vi "Sequencer.vi"() -> ()   [LabVIEW 2014]
uses:
  <vilib>/gmath/statdist.llb/Poisson Random.vi
  <vilib>/Analysis/NI_AALPro.lvlib
  <vilib>/gmath/NI_Gmath.lvlib
panel:
  in  "Ion":bool
  in  "Protect":bool
  out "PMT":dbl=70.0 format="%.1f"
  in  "Experiment":bool
  in  "Pumping":bool
  in  "Detection":bool
  in  "Cooling":bool
  out "History":variant
  in  "Count or State":i16(ring) items=["Count", "State"]
  in  "Channel":string(combo)="c1+c2+c3+c4"
  in  "Device":string(combo)="PMT"
  in  ">":dbl=1.0
  in  "Fit":bool
  out "Peak":u32
  out "Histogram":cluster{"Axis":dbl[], "Histogram":i32[]}(graph)
  in  "Data Chapter":i16(ring) items=["All", "Ion[2]"]
  out "Average Plot":cluster{dbl, dbl}(graph)
  in  "Clear":bool
  in  "Sweep":bool
  in  "Data":bool
  out "data file":string
  in  "Sequence":string
  in  "Chapter (us)":string
  in  "Sequence File":path=path "E:/Data/Sequence/Cooling.seq"
  in  "Repeats":u32=100
  in  "Compile":bool
  in  "Send":bool
  in  "Port":refnum<visa-resource-name>="COM5"
  in  "Trigger":bool
  in  "Save":bool
  out "Item Function":refnum<vi>
  in  "Set":bool
  in  "Item":string(combo)="Time"
  out "SequenceNames":string[](array[string])
  in  "Parameter":u16(ring) items=["Segment", "Frequency", "Duration", "Amplitude", "Phase", "Gap"]
  in  "Scan":bool
  out "Value":dbl=1.0 format="%.4f"
  in  "Step":dbl=1.0 format="%.4f"
  in  "End":dbl=1.0 format="%.3f"
  in  "Start":dbl=1.0 format="%.3f"
  out "Counts":u32[](array[numeric])
  out "CompiledSequence":string="#DopplerCooling\r\n0.9 10100000 00000000 00000000\r\n\r\n#Pump\r\n0.3 01000000 00000000 00000000\r\n\r\n#Pulsed\r\n0.2 00100000 00000000 00000000\r\n0.4 00000100 00000000 00000000\r\n0.2 00000000 10000000 00000000\r\n0.2 01000000 00000000 01000000\n"
  out "ChapterNames":string[](array[string])
  out "ChapterPositions":u32[](array[numeric])
  out "Durations Backup":dbl[](array[numeric])
  out "Durations":dbl[](array[numeric])
  in  "Period (ns)":dbl=5.0
  out "States":string[](array[string])
  in  "Sequencer":bool
  out "Clock":string
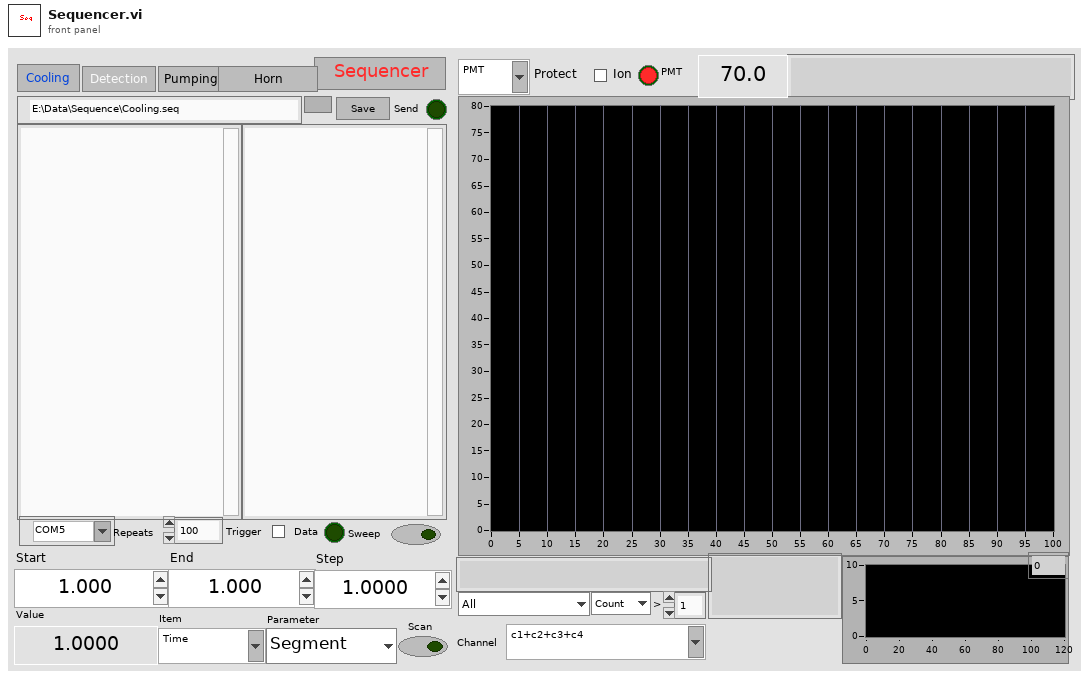
[diagram p1: front panel]
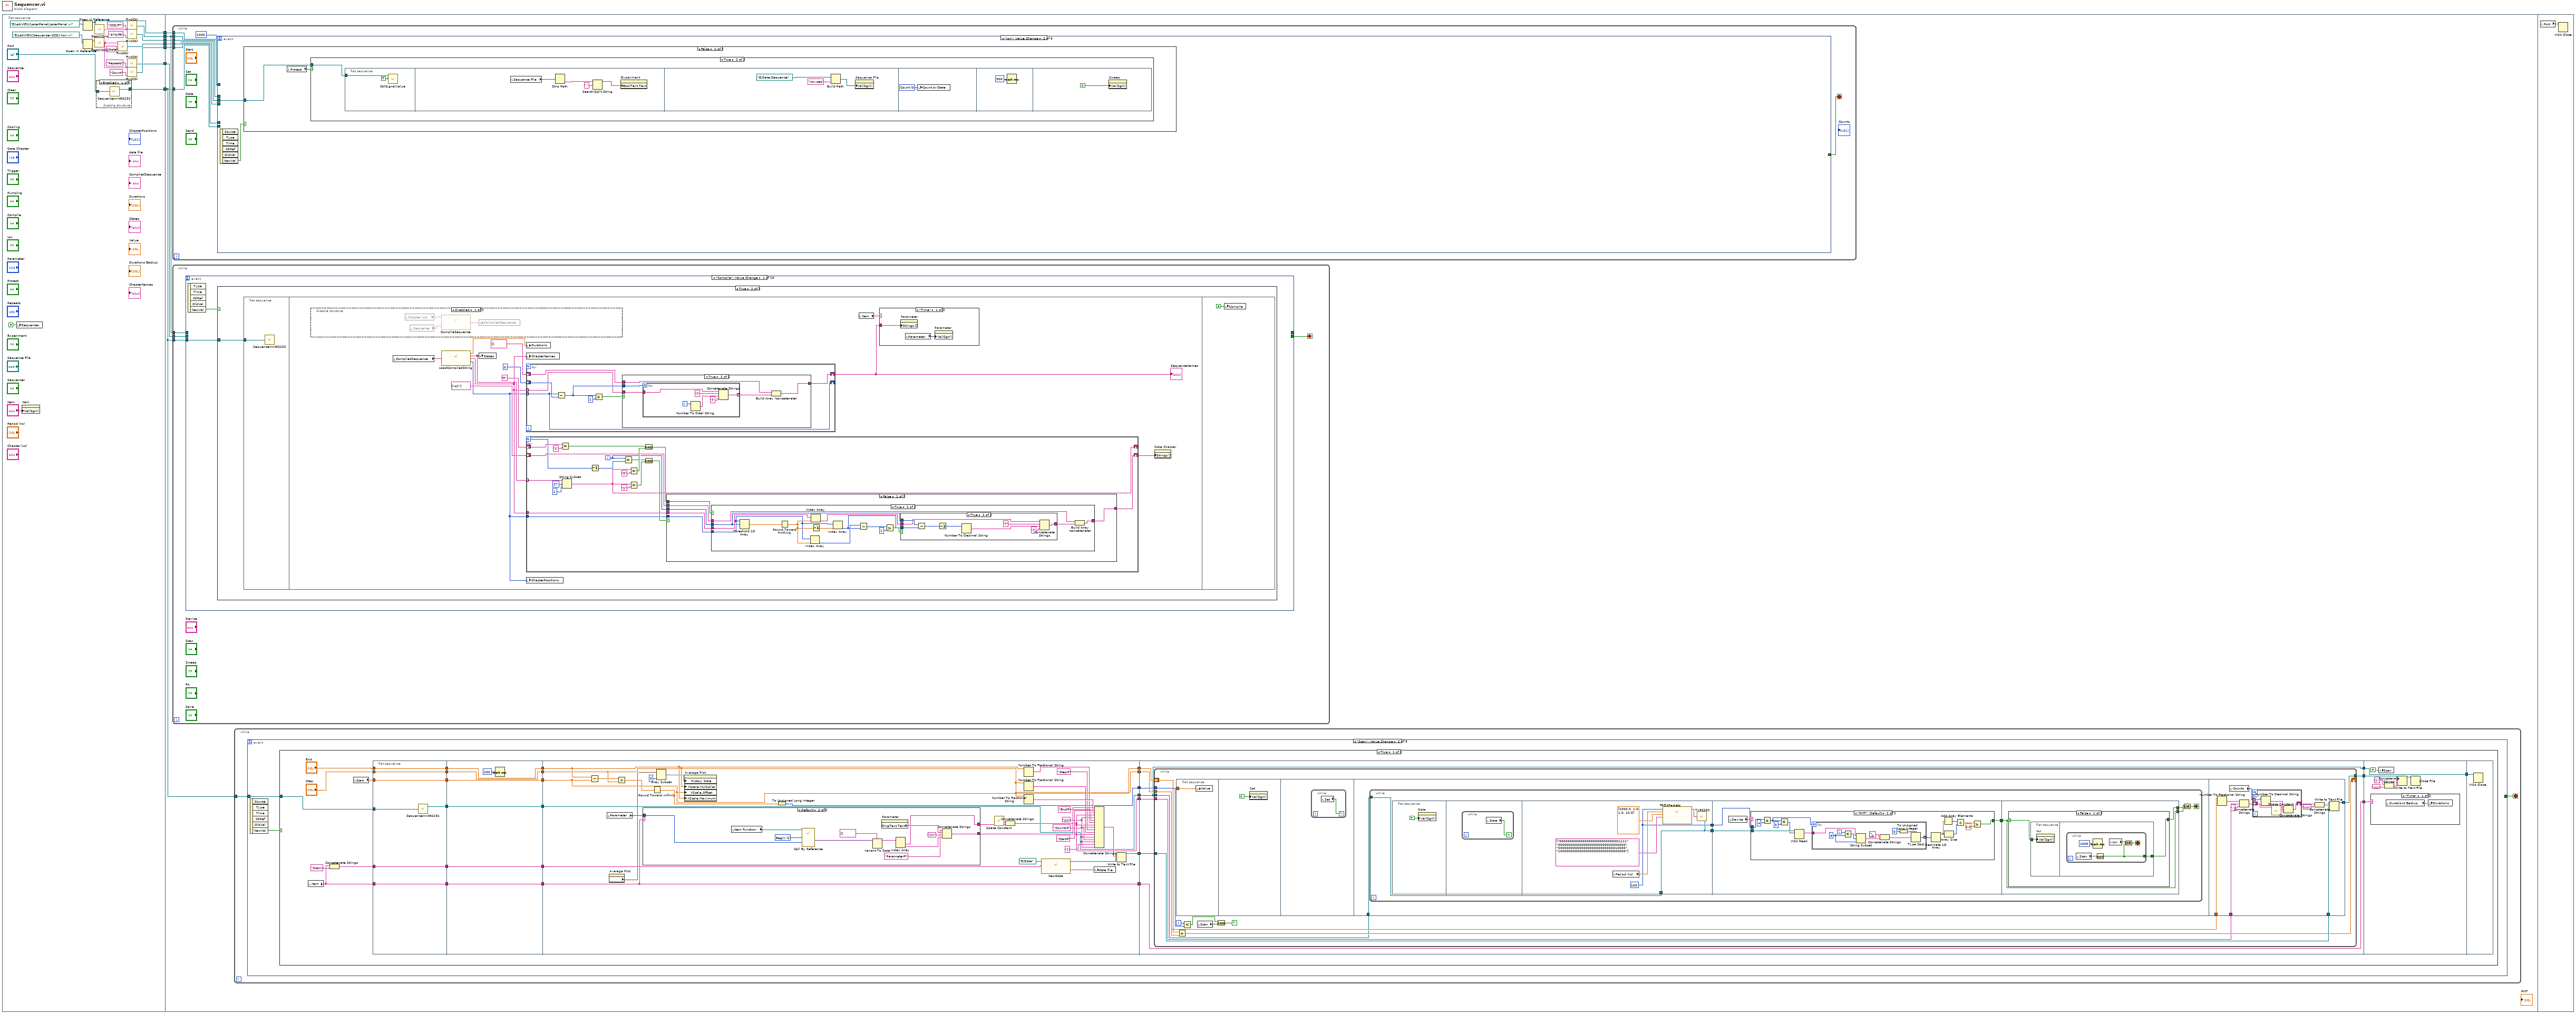
[diagram p0: block diagram]
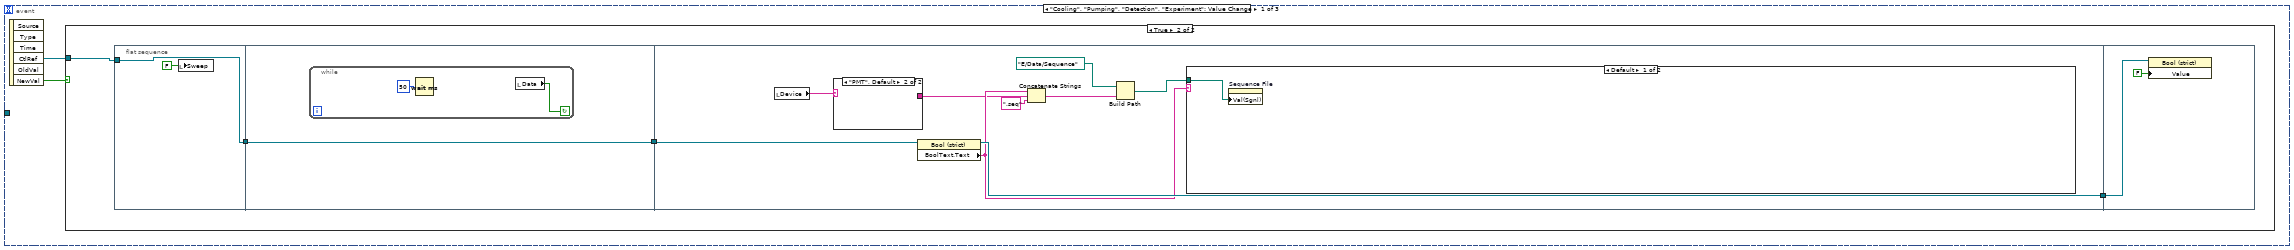
[diagram p3: hidden frame]
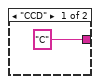
[diagram p5: hidden frame]
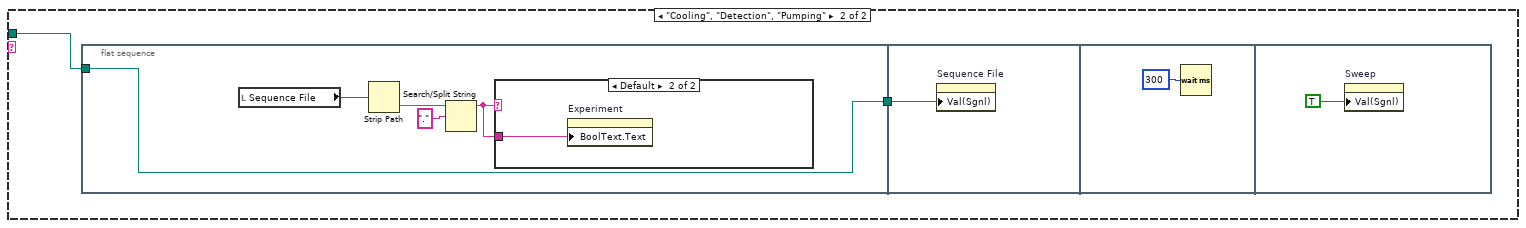
[diagram p6: hidden frame]
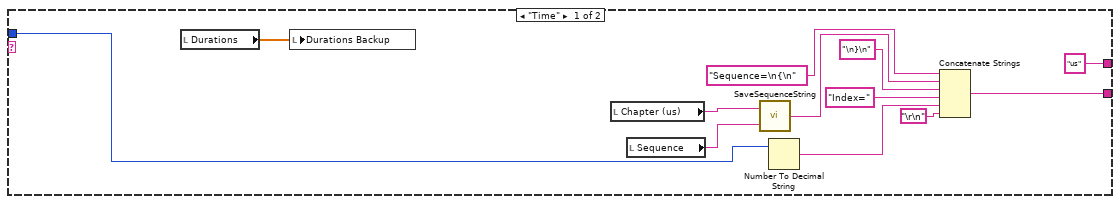
[diagram p8: hidden frame]
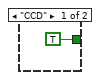
[diagram p9: hidden frame]
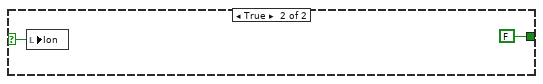
[diagram p10: hidden frame]
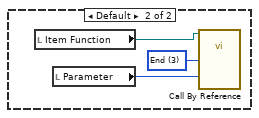
[diagram p11: hidden frame]
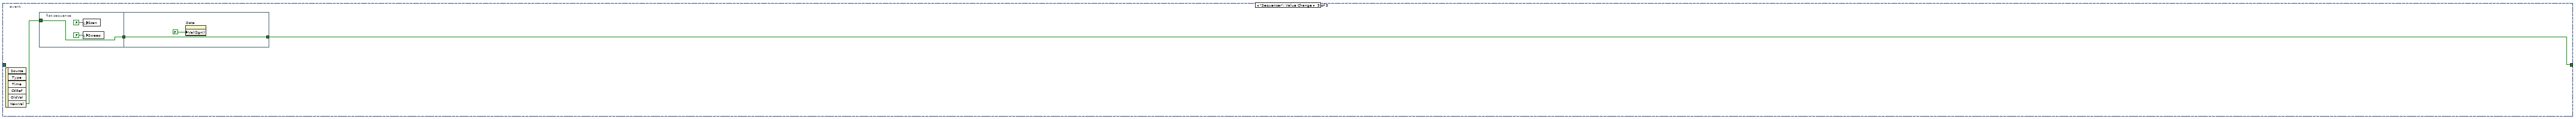
[diagram p13: hidden frame]
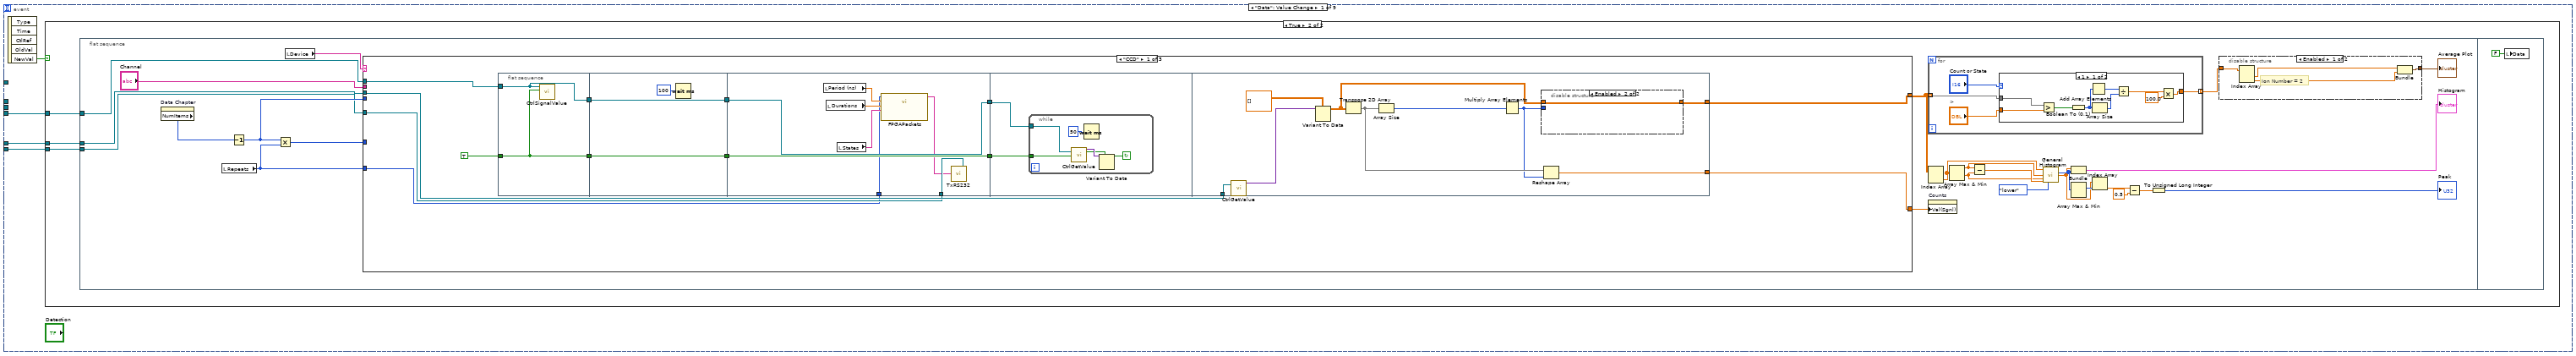
[diagram p14: hidden frame]
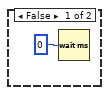
[diagram p15: hidden frame]
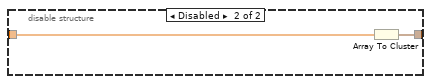
[diagram p16: hidden frame]
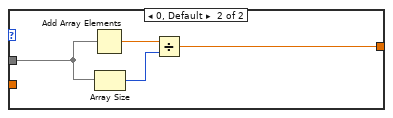
[diagram p17: hidden frame]
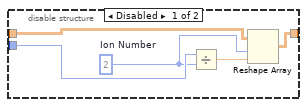
[diagram p18: hidden frame]
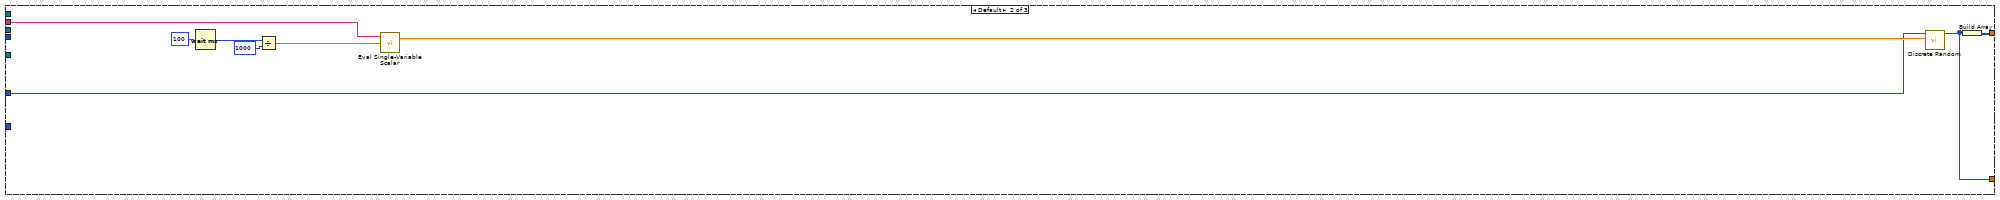
[diagram p19: hidden frame]
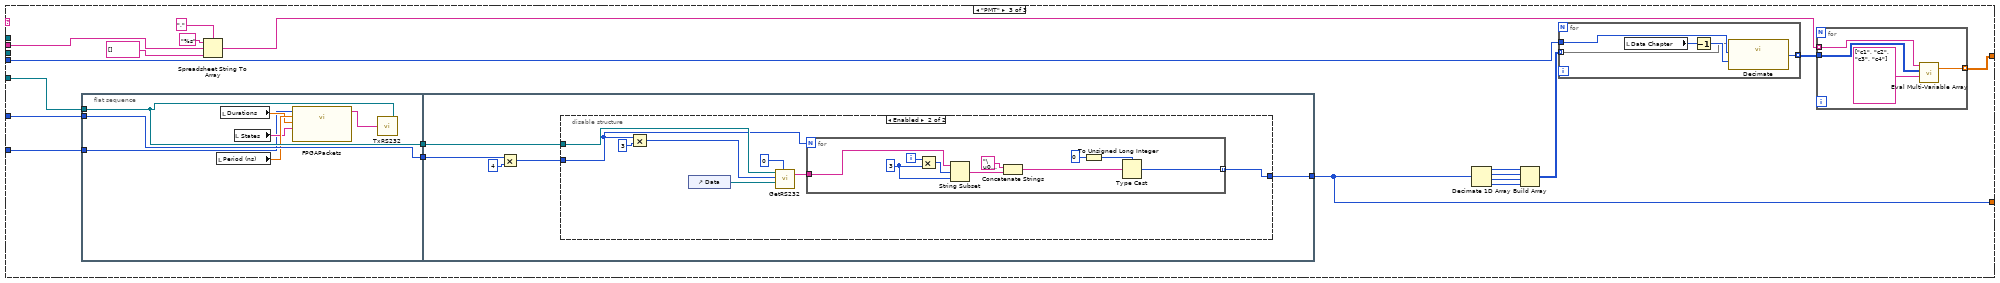
[diagram p20: hidden frame]
diagram:
  n1 = flat-sequence {
    tunnel: [w25] -> w7
    tunnel: [w13] -> w6
    tunnel: [w18] -> w5
    tunnel: [w17] -> w4
    tunnel: [w14] -> w3
    tunnel: [w9] -> w2
    tunnel: [w8] -> w1
    tunnel: w7 -> [w31]
    tunnel: w6 -> [w36]
    tunnel: w5 -> [w35]
    tunnel: w4 -> [w34]
    tunnel: w3 -> [w33]
    tunnel: w2 -> [w30]
    tunnel: w1 -> [w32]
    frame #0 {
      n2 = local write "Sequencer"(FALSE ("Sequencer")) -> ()
      n3 = property on="Item" class="CmbBox"("Val(Sgnl)"="Item") -> ()  [unwired: 2 in, 2 out]
      n4 = Open VI Reference(vi path=path "E:/LabVIEW/LaserPanel/LaserPanel.vi") -> (vi reference=w13:refnum<vi>)  [unwired: 5 in, 1 out]
      n5 = Open VI Reference(vi path=path "E:/LabVIEW/Sequencer.CCD/iXon.vi") -> (vi reference=w21:refnum<vi>)  [unwired: 5 in, 1 out]
      n6 = call "GetAllCtrls.vi"("VI"=w13) -> ("Ctrls"=w11:cluster{"Name":string, "Ctrl":refnum<vi>}[])  [unwired: 1 in]
      n7 = call "GetAllCtrls.vi"("VI"=w21) -> ("Ctrls"=w16:cluster{"Name":string, "Ctrl":refnum<vi>}[])  [unwired: 1 in]
      n8 = disable-structure shown="Enabled" {
        disable-tunnel: "Port" -> [w29 _]
        disable-tunnel: [w28 _] -> w25
        frame Enabled {
          n9 = call "SequencerInitRS232.vi"("VISA resource name"=w29) -> ("reference out"=w28:refnum<visa-resource-name>)  [unwired: 1 out]
        }
        frame Disabled {
        }
      }
      n10 = call "FindCtrl.vi"("Name"="Data", "Ctrls"=w16) -> ("Ctrl"=w18:refnum<vi>)  [unwired: 1 in]
      n11 = call "FindCtrl.vi"("Name"="CCD/F7", "Ctrls"=w11) -> ("Ctrl"=w8:refnum<vi>)  [unwired: 1 in]
      n12 = call "FindCtrl.vi"("Name"="370/F5", "Ctrls"=w11) -> ("Ctrl"=w9:refnum<vi>)  [unwired: 1 in]
      n13 = call "FindCtrl.vi"("Name"="Repeats", "Ctrls"=w16) -> ("Ctrl"=w14:refnum<vi>)  [unwired: 1 in]
      n14 = call "FindCtrl.vi"("Name"="Count", "Ctrls"=w16) -> ("Ctrl"=w17:refnum<vi>)  [unwired: 1 in]
    }
    frame #1 {
      n15 = while {
        tunnel: w31 -> [w301]
        tunnel: w36 -> [w298]
        tunnel: w35 -> [w297]
        tunnel: w34 -> [w296]
        tunnel: w32 -> [w295]
        tunnel: w30 -> [w294]
        stop <- w300 stop-if-true
        n16 = event shown="[1] \"Ion\": Value Change" {
          selector: _ -> [_ _ _ _ _ _ _ _ _]
          dyn-events: _ -> [_ _ _ _ _ _ _ _ _]
          timeout: u32 1000 ("milliseconds to wait") -> [_ _ _ _ _ _ _ _ _]
          tunnel: w301 -> [w305 _ _ _ _ _ _ _ w570]
          tunnel: [_ _ _ _ _ _ _ w569 _] -> w300
          tunnel: w298 -> [_ _ _ _ w544 _ _ _ _]
          tunnel: w297 -> [w303 _ _ _ _ _ _ _ _]
          tunnel: w296 -> [w302 _ _ _ _ _ _ _ _]
          tunnel: w295 -> [_ _ _ w525 _ _ _ _ _]
          tunnel: w294 -> [_ w494 _ _ _ _ _ _ _]
          event "Data": Value Change {
            n17 = event-data() -> ("NewVal"=w304:bool)  [unwired: 1 in, 4 out]
            n18 = case shown="True" w304 {
              tunnel: w305 -> [_ w309]
              tunnel: w303 -> [_ w308]
              tunnel: w302 -> [_ w307]
              frame False {
                n19 = Wait (ms)(milliseconds to wait=u32 0) -> ()  [unwired: 1 out]
              }
              frame True {
                n20 = flat-sequence {
                  tunnel: w308 -> [w312]
                  tunnel: w307 -> [w311]
                  tunnel: w309 -> [w334]
                  frame #0 {
                    n21 = property on="Data Chapter" class="Ring (strict)"() -> ("NumItems"=w333:u32)  [unwired: 2 in, 2 out]
                    n22 = local read "Repeats"() -> (w310:u32)
                    n23 = Decrement(x=w333) -> (x-1=w335:u32)
                    n24 = Multiply(x=w335, y=w310) -> (x*y=w332:u32)
                    n25 = local read "Device"() -> (w313:string)
                    n26 = case shown="\"CCD\"" w313 {
                      tunnel: w335 -> [_ _ w427]
                      tunnel: w334 -> [w364 _ w434]
                      tunnel: w332 -> [_ w414 w433]
                      tunnel: [w367 w413 w432] -> w321
                      tunnel: [w368 w412 w424] -> w315
                      tunnel: "Channel" -> [_ w407 w419]
                      tunnel: w312 -> [w371 _ _]
                      tunnel: w311 -> [w369 _ _]
                      tunnel: w310 -> [w359 _ w416]
                      frame "CCD" {
                        n27 = flat-sequence {
                          tunnel: w371 -> [w373]
                          tunnel: TRUE -> [w372]
                          tunnel: [w373] -> w363
                          tunnel: [w372] -> w361
                          tunnel: w363 -> [w376]
                          tunnel: [w376] -> w362
                          tunnel: w361 -> [w375]
                          tunnel: [w375] -> w360
                          tunnel: w362 -> [w384]
                          tunnel: [w384] -> w366
                          tunnel: w360 -> [w383]
                          tunnel: [w383] -> w365
                          tunnel: w364 -> [w382]
                          tunnel: w359 -> [w377]
                          tunnel: w366 -> [w386]
                          tunnel: w365 -> [w385]
                          tunnel: w369 -> [w400]
                          tunnel: [w394] -> w368
                          tunnel: [w396] -> w367
                          frame #0 {
                            n28 = call "CtrlSignalValue.vi"("variant"=w372, "reference"=w373) -> ()  [unwired: 2 in, 1 out]
                          }
                          frame #1 {
                            n29 = Wait (ms)(milliseconds to wait=u32 100) -> ()  [unwired: 1 out]
                          }
                          frame #2 {
                            n30 = local read "Period (ns)"() -> (w380:dbl)
                            n31 = local read "Durations"() -> (w379:dbl[])
                            n32 = local read "States"() -> (w378:string[])
                            n33 = call "FPGAPackets.vi"("Repeats"=w377, "Period (ns)"=w380, "Durations"=w379, "States"=w378) -> ("Packets"=w381:string)  [unwired: 1 in, 1 out]
                            n34 = call "TxRS232.vi"("VISA resource name"=w382, "Data"=w381) -> ()
                          }
                          frame #3 {
                            n35 = while {
                              tunnel: w386 -> [w390]
                              tunnel: w385 -> [w388]
                              stop <- w387 continue-if-true
                              n36 = call "CtrlGetValue.vi"("reference"=w390) -> ("variant"=w391:variant)  [unwired: 1 in, 3 out]
                              n37 = Wait (ms)(milliseconds to wait=u32 50) -> ()  [unwired: 1 out]
                              n38 = Variant To Data(type=w388, Variant=w391) -> (data=w387:bool)  [unwired: 1 in, 1 out]
                            }
                          }
                          frame #4 {
                            n39 = call "CtrlGetValue.vi"("reference"=w400) -> ("variant"=w399:variant)  [unwired: 1 in, 3 out]
                            n40 = Variant To Data(type=dbl[][] [] ("Count"), Variant=w399) -> (data=w392:dbl[][])  [unwired: 1 in, 1 out]
                            n41 = Transpose 2D Array(2D array=w392) -> (transposed array=w395:dbl[][])
                            n42 = Array Size(array=w395) -> (size(s)=w397:i32[])
                            n43 = Multiply Array Elements(1:w397) -> (0:w393:i32)
                            n44 = disable-structure shown="Enabled" {
                              disable-tunnel: [w405 w406] -> w394
                              disable-tunnel: w393 -> [w404 _]
                              disable-tunnel: w392 -> [w401 w406]
                              frame Disabled {
                                w403 = 2  # Ion Number
                                n45 = Divide(x=w404, y=w403) -> (x/y=w402:dbl)
                                n46 = Reshape Array(w401, w403, w402) -> (w405:dbl[][])
                              }
                              frame Enabled {
                              }
                            }
                            n47 = Reshape Array(w395, w393) -> (w396:dbl[])
                          }
                        }
                      }
                      frame Default {
                        n48 = Wait (ms)(milliseconds to wait=u32 100 ("y")) -> (millisecond timer value=w409:u32)
                        n49 = Divide(x=w409, y=u32 1000) -> (x/y=w411:dbl)
                        n50 = call <vilib>:"Eval Single-Variable Scalar.vi"("x value"=w411, "formula"=w407) -> ("y value"=w415:dbl)  [unwired: 1 in, 1 out]
                        n51 = call-poly <vilib>:"Discrete Random.vi"("lambda"=w415, "samples"=w414) -> ("Poisson random data"=w413:i32[])  [unwired: 8 in, 1 out]
                        n52 = Build Array(w413) -> (w412:i32[][])
                      }
                      frame "PMT" {
                        n53 = flat-sequence {
                          tunnel: w433 -> [w441]
                          tunnel: w434 -> [w440]
                          tunnel: [w440] -> w418
                          tunnel: [w441] -> w417
                          tunnel: w416 -> [w435]
                          tunnel: [w442] -> w432
                          tunnel: w418 -> [w446]
                          tunnel: w417 -> [w445]
                          frame #0 {
                            n54 = local read "Period (ns)"() -> (w438:dbl)
                            n55 = local read "Durations"() -> (w437:dbl[])
                            n56 = local read "States"() -> (w436:string[])
                            n57 = call "FPGAPackets.vi"("Repeats"=w435, "Period (ns)"=w438, "Durations"=w437, "States"=w436) -> ("Packets"=w439:string)  [unwired: 1 in, 1 out]
                            n58 = call "TxRS232.vi"("VISA resource name"=w440, "Data"=w439) -> ()
                          }
                          frame #1 {
                            n59 = Multiply(x=w445, y=u32 4) -> (x*y=w444:u32)
                            n60 = disable-structure shown="Enabled" {
                              disable-tunnel: w446 -> [w449 w471]
                              disable-tunnel: w444 -> [w448 w466]
                              disable-tunnel: [w447 w467] -> w442
                              frame Disabled {
                                n61 = while {
                                tunnel: w449 -> [w461]
                                tunnel: [w462] -> w447 mode=indexing
                                tunnel: w448 -> [w459]
                                i -> [w458]
                                stop <- w464 continue-if-true
                                n62 = Increment(x=w458) -> (x+1=w457:i32)
                                n63 = control-ref of="Data"() -> (w460:refnum<vi>)
                                n64 = Less?(x=w457, y=w459) -> (x < y?=w463:bool)
                                n65 = local read "Data"() -> (w465:bool)
                                n66 = And(x=w463, y=w465) -> (x .and. y?=w464:bool)
                                n67 = call "GetRS232.vi"("VISA resource name"=w461, "Bytes To Read"=3, "Control"=w460, "Limit"=0) -> ("Data"=w451:string)  [unwired: 1 in, 1 out]
                                n68 = Concatenate Strings("\u0000" ("string"), w451) -> (w453:string)
                                n69 = To Unsigned Long Integer(number=u32 0) -> (unsigned 32bit integer=w456:u32)
                                n70 = Type Cast(type=w456, x=w453) -> (*(type *) &x=w462:u32)
                                }
                              }
                              frame Enabled {
                                n71 = Multiply(x=w466, y=3 ("Bytes To Read")) -> (x*y=w470:u32)
                                n72 = control-ref of="Data"() -> (w469:refnum<vi>)
                                n73 = call "GetRS232.vi"("VISA resource name"=w471, "Bytes To Read"=w470, "Control"=w469, "Limit"=0) -> ("Data"=w468:string)  [unwired: 1 in, 1 out]
                                n74 = for {
                                N: w466 -> [_]
                                tunnel: w468 -> [w483]
                                tunnel: [w474] -> w467 mode=indexing
                                i -> [w477]
                                w476 = 3 ("length (rest)")
                                n75 = Multiply(x=w477, y=w476) -> (x*y=w475:i32)
                                n76 = String Subset(string=w483, offset (0)=w475, length (rest)=w476) -> (substring=w478:string)
                                n77 = Concatenate Strings("\u0000" ("string"), w478) -> (w482:string)
                                n78 = To Unsigned Long Integer(number=u32 0) -> (unsigned 32bit integer=w479:u32)
                                n79 = Type Cast(type=w479, x=w482) -> (*(type *) &x=w474:u32)
                                }
                              }
                            }
                          }
                        }
                        n80 = Spreadsheet String To Array(delimiter (Tab)=",", format string="%s", spreadsheet string=w419, array type (2D Dbl)=string[] []) -> (array=w420:string[])
                        n81 = Decimate 1D Array(w432) -> (w431:u32[], w430:u32[], w429:u32[], w428:u32[])
                        n82 = Build Array(w431, w430, w429, w428) -> (w426:u32[][])
                        n83 = for {
                          tunnel: w427 -> [w486]
                          tunnel: w426 -> [w485] mode=indexing
                          tunnel: [w484] -> w425 mode=indexing
                          n84 = local read "Data Chapter"() -> (w487:i16)
                          n85 = Decrement(x=w487) -> (x-1=w488:i16)
                          n86 = call "Decimate.vi"("i"=w488, "n"=w486, "Input Array"=w485) -> ("Decimated Array"=w484:u32[])
                        }
                        n87 = for {
                          tunnel: w425 -> [w492]
                          tunnel: [w490] -> w424 mode=indexing
                          tunnel: w420 -> [w489] mode=indexing
                          n88 = call <vilib>:"Eval Multi-Variable Array.vi"("Variables"=string[] ["c1", "c2", "c3", "c4"], "X Values"=w492, "formula"=w489) -> ("Y Values"=w490:dbl[])  [unwired: 1 in, 1 out]
                        }
                      }
                    }
                    n89 = for {
                      tunnel: w315 -> [w344] mode=indexing
                      tunnel: [w342] -> w318 mode=indexing
                      n90 = case shown="1" "Count or State" {
                        tunnel: [w346 w356] -> w342
                        tunnel: ">" -> [w352 _]
                        tunnel: w344 -> [w351 w355]
                        frame 1 {
                          n91 = Greater?(x=w351, y=w352) -> (0:w353:bool[])
                          n92 = Boolean To (0,1)(Boolean=w353) -> (0, 1=w348:i16[])
                          n93 = Add Array Elements(numeric array=w348) -> (sum=w349:i16)
                          n94 = Array Size(array=w348) -> (size(s)=w350:i32)
                          n95 = Divide(x=w349, y=w350) -> (x/y=w347:dbl)
                          n96 = Multiply(x=w347, y=100.0) -> (x*y=w346:dbl)
                        }
                        frame 0, Default {
                          n97 = Add Array Elements(numeric array=w355) -> (sum=w357:dbl)
                          n98 = Array Size(array=w355) -> (size(s)=w358:i32)
                          n99 = Divide(x=w357, y=w358) -> (x/y=w356:dbl)
                        }
                      }
                    }
                    n100 = Index Array(array=w315) -> (element=w316:dbl[])  [unwired: 2 in]
                    n101 = property on="Counts" class="Arr (strict)"("Val(Sgnl)"=w321) -> ()  [unwired: 2 in, 2 out]
                    n102 = Array Max & Min(array=w316) -> (max value=w330:dbl, min value=w328:dbl)  [unwired: 2 out]
                    n103 = Subtract(x=w330, y=w328) -> (x-y=w329:dbl)
                    n104 = call <vilib>:"General Histogram.vi"("X"=w316, "max"=w330, "min"=w328, "# bins"=w329, "inclusion"=enum32{"lower", "upper"}."lower") -> ("Histogram"=w327:i32[], "Axis"=w325:dbl[])  [unwired: 6 in, 3 out]
                    n105 = Bundle("Axis"=w325, "Histogram"=w327) -> (→"Histogram":cluster{"Axis":dbl[], "Histogram":i32[]})  [unwired: 1 in]
                    n106 = Array Max & Min(array=w327) -> (max index (indices)=w326:i32)  [unwired: 3 out]
                    n107 = Index Array(array=w325, index=w326) -> (element=w323:dbl)
                    n108 = Subtract(x=w323, y=0.5) -> (x-y=w319:dbl)
                    n109 = To Unsigned Long Integer(number=w319) -> (unsigned 32bit integer=→"Peak":u32)
                    n110 = disable-structure shown="Enabled" {
                      disable-tunnel: w318 -> [w338 w341]
                      disable-tunnel: [w337 w340] -> w317
                      frame Enabled {
                        # "Ion Number = 2"
                        n111 = Index Array(array=w338) -> (element #1=w339:dbl, element #2=w336:dbl)  [unwired: 2 in]
                        n112 = Bundle(w339, w336) -> (w337:cluster{dbl, dbl})  [unwired: 1 in]
                      }
                      frame Disabled {
                        n113 = Array To Cluster(array=w341) -> (cluster=w340:cluster{"[0]":dbl, "[1]":dbl})
                      }
                    }
                    "Average Plot" <- w317
                  }
                  frame #1 {
                    n114 = local write "Data"(FALSE ("Acquisition")) -> ()
                  }
                }
              }
            }
          }
          event "Ion": Value Change {
            n115 = event-data() -> ("NewVal"=w495:bool)  [unwired: 1 in, 5 out]
            n116 = case shown="False" w495 {
              tunnel: w494 -> [w496 _]
              frame False {
                n117 = local read "Protect"() -> (w497:bool)
                n118 = case shown="True" w497 {
                  tunnel: w496 -> [_ w498]
                  frame False {
                  }
                  frame True {
                    n119 = flat-sequence {
                      tunnel: w498 -> [w500]
                      frame #0 {
                        n120 = call "CtrlSignalValue.vi"("variant"=TRUE, "reference"=w500) -> ()  [unwired: 2 in, 1 out]
                      }
                      frame #1 {
                        n121 = local read "Sequence File"() -> (w504:path)
                        n122 = Strip Path(path=w504) -> (name=w503:string)  [unwired: 1 out]
                        n123 = Search/Split String(string=w503, search string/char (-)=".") -> (substring before match=w501:string)  [unwired: 1 in, 2 out]
                        n124 = property on="Experiment" class="Bool (strict)"("BoolText.Text"=w501) -> ()  [unwired: 2 in, 2 out]
                      }
                      frame #2 {
                        n125 = Build Path(base path=path "E:/Data/Sequence", name or relative path="Ion.seq" ("string")) -> (appended path=w506:path)
                        n126 = property on="Sequence File" class="Path"("Val(Sgnl)"=w506) -> ()  [unwired: 2 in, 2 out]
                      }
                      frame #3 {
                        w508 = i16 0 items=["Count", "State"] ("Count or State")
                        n127 = local write "Count or State"(w508) -> ()
                      }
                      frame #4 {
                        n128 = Wait (ms)(milliseconds to wait=u32 300) -> ()  [unwired: 1 out]
                      }
                      frame #5 {
                        n129 = property on="Sweep" class="Bool (strict)"("Val(Sgnl)"=TRUE ("Value (Signaling)")) -> ()  [unwired: 2 in, 2 out]
                      }
                    }
                  }
                }
              }
              frame True {
              }
            }
          }
          event "Set": Value Change {
            n130 = event-data() -> ("NewVal"=w511:bool)  [unwired: 1 in, 5 out]
            n131 = case shown="True" w511 {
              frame False {
              }
              frame True {
                n132 = flat-sequence {
                  frame #0 {
                    n133 = local read "Value"() -> (w512:dbl)
                    n134 = local read "Item"() -> (w513:string)
                    n135 = case shown="Default" w513 {
                      tunnel: w512 -> [w514 w520]
                      frame "Time" {
                        n136 = local read "Parameter"() -> (w517:u16)
                        n137 = local read "Durations"() -> (w515:dbl[])
                        n138 = Replace Array Subset(array=w515, new element=w514, index=w517) -> (w516:dbl[])
                        n139 = local write "Durations"(w516) -> ()
                      }
                      frame Default {
                        w521 = u32 5 items=["Open", "Close", "Begin", "End", "Get", "Set"] ("Mode")
                        n140 = local read "Parameter"() -> (w519:u16)
                        n141 = local read "Item Function"() -> (w522:refnum<vi>)
                        n142 = Build Array(w520, w519) -> (w518:dbl[])
                        n143 = call-by-ref "?"(reference=w522, "In"=w518, "Mode"=w521) -> ()  [unwired: 1 in, 3 out]
                      }
                    }
                  }
                  frame #1 {
                    n144 = local write "Set"(FALSE ("Ready")) -> ()
                  }
                }
              }
            }
          }
          event "Device": Value Change {
            w529 = 2  # Ion Number
            n145 = event-data() -> ("NewVal"=w526:string)  [unwired: 1 in, 5 out]
            n146 = case shown="\"PMT\", Default" w526 {
              tunnel: w525 -> [w538 w541]
              tunnel: [w537 w540] -> w527
              tunnel: [1 260] -> w524
              frame "PMT", Default {
                w537 = FALSE
                n147 = call "CtrlSignalValue.vi"("variant"=w537, "reference"=w538) -> ()  [unwired: 2 in, 1 out]
              }
              frame "CCD" {
                w540 = TRUE
                n148 = call "CtrlSignalValue.vi"("variant"=w540, "reference"=w541) -> ()  [unwired: 2 in, 1 out]
              }
            }
            n149 = case shown="\"Test\"" w526 {
              tunnel: [_ "c1+c2+c3+c4" "10*sin(x)^2"] -> w530
              frame Default {
              }
              frame "PMT" {
              }
              frame "Test" {
              }
            }
            n150 = local write ">"(w524) -> ()
            n151 = Decrement(x=w529) -> (x-1=w528:i32)
            n152 = for {
              N: w528 -> [_]
              tunnel: w527 -> [w533]
              i -> [w532]
              n153 = Increment(x=w532) -> (x+1=w531:i32)
              n154 = property on="Average Plot" class="WFChart (strict)"("Active Plot"=w531, "Plot.Visible?"=w533) -> ("DigDisps[]"=w534:refnum<vi>[])  [unwired: 2 in, 2 out]
              n155 = Index Array(array=w534, index=w531) -> (element=w535:refnum<vi>)
              n156 = property class="DigNum"(reference=w535, "Visible"=w533) -> ()  [unwired: 1 in, 2 out]
            }
            n157 = local write "Channel"(w530) -> ()
          }
          event Timeout {
            n158 = event-data() -> ()  [unwired: 1 in, 3 out]
            n159 = local read "Sweep"() -> (w547:bool)
            n160 = local read "Scan"() -> (w546:bool)
            n161 = Or(x=w547, y=w546) -> (x .or. y?=w545:bool)
            n162 = case shown="False" w545 {
              tunnel: w544 -> [w560 _]
              frame False {
                n163 = invoke class="VI" method="Ctrl Val.Get"(reference=w560, "Control Name"="PMT") -> (reference out=w557:refnum<vi>, "Get Control Value Variant"=w562:variant)  [unwired: 2 in, 2 out]
                n164 = Variant To Data(type=0.0, Variant=w562) -> (data=w559:dbl)  [unwired: 1 in, 1 out]
                n165 = invoke class="VI" method="Ctrl Val.Get"(reference=w557, "Control Name"="CCD/F7" ("Name")) -> ("Get Control Value Variant"=w555:variant)  [unwired: 2 in, 3 out]
                n166 = local write "PMT"(w559) -> ()
                n167 = Variant To Data(type=FALSE, Variant=w555) -> (data=w553:bool)  [unwired: 1 in, 1 out]
                n168 = Greater?(x=w559, y=20.0) -> (0:w552:bool)
                n169 = Or(x=w553, y=w552) -> (x .or. y?=w551:bool)
                n170 = property on="Ion" class="Bool (strict)"("Val(Sgnl)"=w551) -> ()  [unwired: 2 in, 2 out]
              }
              frame True {
              }
            }
            n171 = Get Date/Time In Seconds() -> (seconds since 1Jan1904=w548:timestamp)
            n172 = Format Date/Time String(time format string (%c)="%Y/%m/%d %H:%M:%S", seconds (now)=w548) -> (date/time string=→"Clock":string)  [unwired: 1 in]
          }
          event "Protect": Value Change {
            n173 = event-data() -> ("NewVal"=w564:bool)  [unwired: 1 in, 5 out]
            n174 = case shown="True" w564 {
              frame False {
              }
              frame True {
                n175 = local read "Ion"() -> (w565:bool)
                n176 = property on="Ion" class="Bool (strict)"("Val(Sgnl)"=w565) -> ()  [unwired: 2 in, 2 out]
              }
            }
          }
          event "Start": Value Change {
            n177 = event-data() -> ("NewVal"=w566:dbl)  [unwired: 1 in, 5 out]
            n178 = flat-sequence {
              tunnel: w566 -> [w567]
              frame #0 {
                n179 = local write "Value"(w567) -> ()
              }
              frame #1 {
                n180 = property on="Set" class="Bool (strict)"("Val(Sgnl)"=TRUE ("Value (Signaling)")) -> ()  [unwired: 2 in, 2 out]
              }
            }
          }
          event "Sequencer": Value Change {
            n181 = event-data() -> ("NewVal"=w569:bool)  [unwired: 1 in, 4 out]
          }
          event "Send": Value Change {
            n182 = event-data() -> ("NewVal"=w571:bool)  [unwired: 1 in, 4 out]
            n183 = case shown="True" w571 {
              tunnel: w570 -> [_ w572]
              frame False {
              }
              frame True {
                n184 = flat-sequence {
                  tunnel: w572 -> [w573]
                  frame #0 {
                    n185 = local read "Period (ns)"() -> (w577:dbl)
                    n186 = local read "Durations"() -> (w575:dbl[])
                    n187 = local read "Repeats"() -> (w576:u32)
                    n188 = local read "States"() -> (w578:string[])
                    n189 = call "FPGAPackets.vi"("Repeats"=w576, "Period (ns)"=w577, "Durations"=w575, "States"=w578) -> ("Packets"=w574:string)  [unwired: 1 in, 1 out]
                    n190 = call "TxRS232.vi"("VISA resource name"=w573, "Data"=w574) -> ()
                  }
                  frame #1 {
                    n191 = local write "Send"(FALSE ("Send")) -> ()
                  }
                }
              }
            }
          }
        }
      }
      n192 = while {
        tunnel: w33 -> [w582]
        tunnel: w32 -> [w581]
        tunnel: w31 -> [w580]
        stop <- w583 stop-if-true
        n193 = event shown="[0] \"Compile\": Value Change" {
          selector: _ -> [_ _ _ _ _ _ _ _ _ _]
          dyn-events: _ -> [_ _ _ _ _ _ _ _ _ _]
          timeout: _ -> [_ _ _ _ _ _ _ _ _ _]
          tunnel: [_ _ _ _ _ _ _ _ _ w803] -> _
          tunnel: [_ _ _ _ _ _ _ _ _ w803] -> w583
          tunnel: w582 -> [_ _ _ _ _ _ _ w772 _ _]
          tunnel: w581 -> [_ _ _ _ _ _ _ _ _ _]
          tunnel: w580 -> [w584 _ _ _ _ _ _ _ w778 _]
          event "Compile": Value Change {
            n194 = event-data() -> ("NewVal"=w585:bool)  [unwired: 1 in, 4 out]
            n195 = case shown="True" w585 {
              tunnel: w584 -> [_ w586]
              frame False {
              }
              frame True {
                n196 = flat-sequence {
                  tunnel: w586 -> [w587]
                  frame #0 {
                    n197 = call "SequencerInitRS232.vi"("VISA resource name"=w587) -> ()  [unwired: 2 out]
                  }
                  frame #1 {
                    n198 = disable-structure shown="Disabled" {
                      frame Disabled {
                        n199 = local read "Chapter (us)"() -> (w604:string)
                        n200 = local read "Sequence"() -> (w603:string)
                        n201 = call "CompileSequence.vi"("Sequence"=w603, "Chapter"=w604) -> ("Compiled Sequence"=w602:string)
                        n202 = local write "CompiledSequence"(w602) -> ()
                      }
                      frame Enabled {
                      }
                    }
                    n203 = local read "CompiledSequence"() -> (w590:string)
                    n204 = call "LoadCompiledString.vi"("Compiled String"=w590) -> ("Durations"=w599:dbl[], "States"=w598:string[], "ChapterNames"=w591:string[], "ChapterPositions"=w592:u32[])
                    n205 = local write "States"(w598) -> ()
                    n206 = local write "Durations"(w599) -> ()
                    n207 = local write "ChapterNames"(w591) -> ()
                    n208 = for {
                      tunnel: w592 -> [w605] mode=indexing
                      tunnel: w591 -> [w606] mode=indexing
                      shift-right: [w605] -> _
                      shift-left: u32 0 ("initial scan location") -> [w612]
                      shift-right: [w607] -> w588
                      shift-left: string[] [] -> [w608]
                      n209 = Subtract(x=w605, y=w612) -> (x-y=w609:u32)
                      n210 = Greater?(x=w609, y=u32 1) -> (0:w611:bool)
                      n211 = case shown="True" w611 {
                        tunnel: w606 -> [w614 w620]
                        tunnel: w609 -> [_ w619]
                        tunnel: w608 -> [w615 w618]
                        tunnel: [w613 w616] -> w607
                        frame False {
                          n212 = Build Array (concatenate)(w615, w614) -> (w613:string[])
                        }
                        frame True {
                          n213 = for {
                            N: w619 -> [_]
                            tunnel: w620 -> [w625]
                            tunnel: [w624] -> w617 mode=indexing
                            i -> [w626]
                            n214 = Number To Octal String(2:w626) -> (0:w623:string)  [unwired: 1 in]
                            n215 = Concatenate Strings(w625, "[" ("string"), w623, "]" ("string")) -> (w624:string)
                          }
                          n216 = Build Array (concatenate)(w618, w617) -> (w616:string[])
                        }
                      }
                    }
                    "SequenceNames" <- w588
                    n217 = for {
                      N -> [w638]
                      tunnel: w598 -> [w647] mode=indexing
                      shift-right: [w635] -> _
                      shift-left: "0" -> [w645]
                      tunnel: w591 -> [w641]
                      shift-right: [w630] -> w594
                      shift-left: string[] ["All"] -> [w629]
                      tunnel: w592 -> [w628]
                      i -> [w639]
                      n218 = Equal?(x=w645, y="1") -> (x = y?=w643:bool)
                      n219 = String Subset(string=w647, offset (0)=27, length (rest)=1 ("length (rest)")) -> (substring=w635:string)
                      n220 = Decrement(x=w638) -> (x-1=w637:i32)
                      n221 = Equal?(x=w639, y=w637) -> (x = y?=w634:bool)
                      n222 = Equal?(x=w635, y="0") -> (x = y?=w640:bool)
                      n223 = Equal?(x=w635, y="1") -> (x = y?=w633:bool)
                      n224 = And(x=w643, y=w640) -> (x .and. y?=w631:bool)
                      n225 = And(x=w634, y=w633) -> (x .and. y?=w632:bool)
                      n226 = case shown="False" w632 {
                        tunnel: w641 -> [w653 w693]
                        tunnel: w629 -> [w652 w695]
                        tunnel: w639 -> [w651 _]
                        tunnel: w631 -> [w650 _]
                        tunnel: [w649 w694] -> w630
                        tunnel: w628 -> [w648 w687]
                        frame False {
                          n227 = case shown="True" w650 {
                            tunnel: w651 -> [_ w665]
                            tunnel: w653 -> [_ w666]
                            tunnel: w652 -> [w654 w668]
                            tunnel: [w654 w669] -> w649
                            tunnel: w648 -> [_ w662]
                            frame False {
                            }
                            frame True {
                              n228 = Threshold 1D Array(2:w665, 3:w662) -> (0:w667:dbl)  [unwired: 1 in]
                              n229 = Round Toward +Infinity(x=w667) -> (ceil(x): smallest int >= x=w660:dbl)
                              n230 = Index Array(array=w662, index=w660) -> (element=w659:u32)
                              n231 = Index Array(array=w666, index=w660) -> (element=w663:string)
                              n232 = Decrement(x=w660) -> (x-1=w661:dbl)
                              n233 = Index Array(array=w662, index=w661) -> (element=w655:u32)
                              n234 = Subtract(x=w659, y=w655) -> (x-y=w658:u32)
                              n235 = Greater?(x=w658, y=u32 1) -> (0:w656:bool)
                              n236 = case shown="True" w656 {
                                tunnel: w665 -> [_ w679]
                                tunnel: [w670 w673] -> w664
                                tunnel: w663 -> [w670 w672]
                                tunnel: w655 -> [_ w671]
                                frame False {
                                }
                                frame True {
                                n237 = Subtract(x=w679, y=w671) -> (x-y=w678:u32)
                                n238 = Decrement(x=w678) -> (x-1=w677:u32)
                                n239 = Number To Decimal String(number=w677) -> (decimal integer string=w674:string)  [unwired: 1 in]
                                n240 = Concatenate Strings(w672, "[" ("element"), w674, "]" ("element")) -> (w673:string)
                                }
                              }
                              n241 = Build Array (concatenate)(w668, w664) -> (w669:string[])
                            }
                          }
                        }
                        frame True {
                          n242 = Array Size(array=w693) -> (size(s)=w692:i32)
                          n243 = Array Size(array=w687) -> (size(s)=w690:i32)
                          n244 = Decrement(x=w692) -> (x-1=w691:i32)
                          n245 = Decrement(x=w690) -> (x-1=w689:i32)
                          n246 = Index Array(array=w687, index=w689) -> (element=w686:u32)
                          n247 = Index Array(array=w693, index=w691) -> (element=w682:string)
                          n248 = Decrement(x=w689) -> (x-1=w688:i32)
                          n249 = Index Array(array=w687, index=w688) -> (element=w685:u32)
                          n250 = Subtract(x=w686, y=w685) -> (x-y=w680:u32)
                          n251 = Greater?(x=w680, y=u32 1) -> (0:w683:bool)
                          n252 = case shown="True" w683 {
                            tunnel: w682 -> [w696 w703]
                            tunnel: [w696 w697] -> w681
                            tunnel: w680 -> [_ w700]
                            frame False {
                            }
                            frame True {
                              n253 = Decrement(x=w700) -> (x-1=w699:u32)
                              n254 = Number To Octal String(2:w699) -> (0:w698:string)  [unwired: 1 in]
                              n255 = Concatenate Strings(w703, "[" ("string"), w698, "]" ("string")) -> (w697:string)
                            }
                          }
                          n256 = Build Array (concatenate)(w695, w681) -> (w694:string[])
                        }
                      }
                    }
                    n257 = local write "ChapterPositions"(w592) -> ()
                    n258 = local read "Item"() -> (w589:string)
                    n259 = case shown="\"Time\"" w589 {
                      tunnel: w588 -> [w601 _]
                      frame "Time" {
                        n260 = property on="Parameter" class="Ring (strict)"("Strings []"=w601) -> ()  [unwired: 2 in, 2 out]
                        n261 = local read "Parameter"() -> (w600:u16)
                        n262 = property on="Parameter" class="Ring (strict)"("Val(Sgnl)"=w600) -> ()  [unwired: 2 in, 2 out]
                      }
                      frame Default {
                      }
                    }
                    n263 = property on="Data Chapter" class="Ring (strict)"("Strings []"=w594) -> ()  [unwired: 2 in, 2 out]
                  }
                  frame #2 {
                    n264 = local write "Compile"(FALSE ("Compile")) -> ()
                  }
                }
              }
            }
          }
          event "Item": Value Change {
            n265 = event-data() -> ("NewVal"=w706:string)  [unwired: 1 in, 5 out]
            n266 = flat-sequence {
              tunnel: w706 -> [w710]
              tunnel: [w710] -> w705
              tunnel: w705 -> [w712]
              frame #0 {
                w709 = u32 1 items=["Open", "Close", "Begin", "End", "Get", "Set"] ("Mode")
                n267 = local read "Item Function"() -> (w708:refnum<vi>)
                n268 = call-by-ref "?"(reference=w708, "Mode"=w709) -> (error out=w707:errorcluster)  [unwired: 2 in, 2 out]
                n269 = call <vilib>:"Clear Errors.vi"("error in (no error)"=w707) -> ()  [unwired: 5 in, 2 out]
              }
              frame #1 {
                n270 = case shown="Default" w712 {
                  selector: w712 -> [w720 _]
                  tunnel: [w713 w725] -> w711
                  frame Default {
                    w716 = u32 0 items=["Open", "Close", "Begin", "End", "Get", "Set"] ("Mode")
                    n271 = Concatenate Strings(w720, ".vi" ("string")) -> (w718:string)
                    n272 = Current VI's Path() -> (path=w722:path)
                    n273 = Strip Path(path=w722) -> (stripped path=w721:path)  [unwired: 1 out]
                    n274 = Build Path(base path=w721, name or relative path=w718) -> (appended path=w723:path)
                    n275 = Open VI Reference(type specifier VI Refnum (for type only)=refnum<vi> refnum, vi path=w723) -> (vi reference=w717:refnum<vi>)  [unwired: 4 in, 1 out]
                    "Item Function" <- w717
                    n276 = call-by-ref "?"(reference=w717, "Mode"=w716) -> ("Out"=w715:variant)  [unwired: 2 in, 2 out]
                    n277 = Variant To Data(type=string[] [] ("Strings []"), Variant=w715) -> (data=w713:string[])  [unwired: 1 in, 1 out]
                  }
                  frame "Time" {
                    n278 = local read "SequenceNames"() -> (w725:string[])
                  }
                }
                n279 = property on="Parameter" class="Ring (strict)"("Strings []"=w711) -> ()  [unwired: 2 in, 2 out]
              }
              frame #2 {
                n280 = disable-structure shown="Enabled" {
                  disable-tunnel: [w727 u16 0 ("Parameter")] -> w726
                  frame Disabled {
                    n281 = local read "Parameter"() -> (w727:u16)
                  }
                  frame Enabled {
                  }
                }
                n282 = property on="Parameter" class="Ring (strict)"("Val(Sgnl)"=w726) -> ()  [unwired: 2 in, 2 out]
              }
            }
          }
          event "Parameter": Value Change {
            n283 = event-data() -> ("NewVal"=w729:u16)  [unwired: 1 in, 5 out]
            n284 = local read "Item"() -> (w731:string)
            n285 = case shown="Default" w731 {
              tunnel: [w733 w736] -> w730
              tunnel: w729 -> [w732 w735]
              frame "Time" {
                n286 = local read "Durations"() -> (w734:dbl[])
                n287 = Index Array(array=w734, index=w732) -> (element=w733:dbl)
              }
              frame Default {
                w739 = u32 4 items=["Open", "Close", "Begin", "End", "Get", "Set"] ("Mode")
                n288 = local read "Item Function"() -> (w740:refnum<vi>)
                n289 = call-by-ref "?"(reference=w740, "In"=w735, "Mode"=w739) -> ("Out"=w738:variant)  [unwired: 1 in, 2 out]
                n290 = Variant To Data(type=0.0, Variant=w738) -> (data=w736:dbl)  [unwired: 1 in, 1 out]
              }
            }
            n291 = local write "Value"(w730) -> ()
          }
          event "Save": Value Change {
            n292 = event-data() -> ("NewVal"=w741:bool)  [unwired: 1 in, 4 out]
            n293 = case shown="True" w741 {
              frame False {
              }
              frame True {
                n294 = flat-sequence {
                  frame #0 {
                    n295 = local read "Sequence File"() -> (w746:path)
                    n296 = local read "Chapter (us)"() -> (w744:string)
                    n297 = local read "Sequence"() -> (w743:string)
                    n298 = call "SaveSequenceString.vi"("Sequence"=w743, "Chapter"=w744) -> ("Sequence String"=w745:string)
                    n299 = call "CompileSequence.vi"("Sequence"=w743, "Chapter"=w744) -> ("Compiled Sequence"=w742:string)
                    n300 = Not Equal?(x=w746, y=path "") -> (x != y?=w748:bool)
                    n301 = case shown="True" w748 {
                      tunnel: w746 -> [_ w750]
                      tunnel: w745 -> [_ w749]
                      frame False {
                      }
                      frame True {
                        n302 = Write to Text File(file (use dialog)=w750, text=w749) -> ()  [unwired: 2 in, 3 out]
                      }
                    }
                    n303 = local write "CompiledSequence"(w742) -> ()
                  }
                  frame #1 {
                    n304 = local write "Save"(FALSE ("Compile")) -> ()
                    n305 = property on="Compile" class="Bool (strict)"("Val(Sgnl)"=TRUE ("Value (Signaling)")) -> ()  [unwired: 2 in, 2 out]
                  }
                }
              }
            }
          }
          event "Fit": Value Change {
            n306 = event-data() -> ("NewVal"=w753:bool)  [unwired: 1 in, 4 out]
            n307 = case shown="True" w753 {
              frame False {
              }
              frame True {
                n308 = local write "Fit"(FALSE ("Fit")) -> ()
                n309 = property on="Average Plot" class="WFChart (strict)"() -> ("History Data"=w755:cluster{dbl, dbl}[])  [unwired: 2 in, 2 out]
                n310 = To Variant(anything=w755) -> (Variant=→"History":variant)
              }
            }
          }
          event "Clear": Value Change {
            n311 = event-data() -> ()  [unwired: 1 in, 6 out]
            n312 = property on="Average Plot" class="WFChart (strict)"() -> ("History Data"=w759:cluster{dbl, dbl}[])  [unwired: 2 in, 2 out]
            n313 = Array Subset(array=w759, length=0) -> (w758:cluster{dbl, dbl}[])  [unwired: 1 in]
            n314 = property on="Average Plot" class="WFChart (strict)"("History Data"=w758) -> ()  [unwired: 2 in, 2 out]
          }
          event "Sequence File": Value Change {
            n315 = event-data() -> ("NewVal"=w761:path)  [unwired: 1 in, 4 out]
            n316 = call <vilib>:"Check if File or Folder Exists.vi"("path"=w761) -> ("file or folder exists?"=w762:bool, "dup path"=w760:path)  [unwired: 8 in, 1 out]
            n317 = case shown="True" w762 {
              tunnel: w760 -> [_ w763]
              frame False {
              }
              frame True {
                n318 = flat-sequence {
                  tunnel: w763 -> [w767]
                  frame #0 {
                    n319 = Read from Text File(file (use dialog)=w767) -> (text=w768:string)  [unwired: 3 in, 3 out]
                    n320 = call "LoadSequenceString.vi"("Sequence String"=w768) -> ("Chapter"=w766:string, "Sequence"=w765:string)
                    n321 = local write "Chapter (us)"(w766) -> ()
                    n322 = call "CompileSequence.vi"("Sequence"=w765, "Chapter"=w766) -> ("Compiled Sequence"=w764:string)
                    n323 = local write "Sequence"(w765) -> ()
                    n324 = local write "CompiledSequence"(w764) -> ()
                  }
                  frame #1 {
                    n325 = property on="Compile" class="Bool (strict)"("Val(Sgnl)"=TRUE ("Value (Signaling)")) -> ()  [unwired: 2 in, 2 out]
                  }
                }
              }
            }
          }
          event "Repeats": Value Change {
            n326 = event-data() -> ("NewVal"=w771:u32)  [unwired: 1 in, 5 out]
            n327 = local read "Device"() -> (w770:string)
            n328 = case shown="\"CCD\"" w770 {
              tunnel: w772 -> [_ w777]
              tunnel: w771 -> [_ w774]
              frame "PMT", Default {
              }
              frame "CCD" {
                n329 = property on="Data Chapter" class="Ring (strict)"() -> ("NumItems"=w776:u32)  [unwired: 2 in, 2 out]
                n330 = Decrement(x=w776) -> (x-1=w775:u32)
                n331 = Multiply(x=w775, y=w774) -> (x*y=w773:u32)
                n332 = call "CtrlSignalValue.vi"("variant"=w773, "reference"=w777) -> ()  [unwired: 2 in, 1 out]
              }
            }
          }
          event "Sweep": Value Change {
            n333 = event-data() -> ("NewVal"=w779:bool)  [unwired: 1 in, 4 out]
            n334 = case shown="True" w779 {
              tunnel: w778 -> [_ w784]
              frame False {
              }
              frame True {
                n335 = flat-sequence {
                  tunnel: w784 -> [w786]
                  tunnel: [w785] -> w781
                  tunnel: w781 -> [w788]
                  tunnel: [w788] -> w780
                  tunnel: [w789] -> w783
                  tunnel: w780 -> [w789]
                  tunnel: w783 -> [w798]
                  tunnel: [w798] -> w782
                  tunnel: w782 -> [w802]
                  frame #0 {
                    n336 = call "SequencerInitRS232.vi"("VISA resource name"=w786) -> ("reference out"=w785:refnum<visa-resource-name>)  [unwired: 1 out]
                  }
                  frame #1 {
                    n337 = Wait (ms)(milliseconds to wait=u32 200) -> ()  [unwired: 1 out]
                  }
                  frame #2 {
                    n338 = local write "data file"("") -> ()
                    n339 = property on="Average Plot" class="WFChart (strict)"() -> ("History Data"=w792:cluster{dbl, dbl}[])  [unwired: 2 in, 2 out]
                    n340 = Array Subset(array=w792, length=0) -> (w790:cluster{dbl, dbl}[])  [unwired: 1 in]
                    n341 = property on="Average Plot" class="WFChart (strict)"("History Data"=w790) -> (error out=w794:errorcluster)  [unwired: 2 in, 1 out]
                    n342 = property on="Average Plot" class="WFChart (strict)"(error in=w794, "XScale.Multiplier"=1.0 ("X Scale.Offset and Multiplier:Multiplier"), "XScale.Offset"=0.0 ("X Scale.Offset and Multiplier:Offset"), "XScale.Maximum"=100.0 ("X Scale.Range:Maximum")) -> ()  [unwired: 1 in, 2 out]
                  }
                  frame #3 {
                    n343 = while {
                      stop <- w799 continue-if-true
                      n344 = flat-sequence {
                        frame #0 {
                          n345 = property on="Data" class="Bool (strict)"("Val(Sgnl)"=TRUE ("Value (Signaling)")) -> ()  [unwired: 2 in, 2 out]
                        }
                        frame #1 {
                          n346 = while {
                            stop <- w801 continue-if-true
                            n347 = local read "Data"() -> (w801:bool)
                          }
                        }
                      }
                      n348 = local read "Sweep"() -> (w799:bool)
                    }
                  }
                  frame #4 {
                    n349 = VISA Close(VISA resource name=w802) -> ()  [unwired: 1 in, 1 out]
                  }
                }
              }
            }
          }
          event "Sequencer": Value Change {
            n350 = event-data() -> ("NewVal"=w803:bool)  [unwired: 1 in, 4 out]
          }
        }
      }
      n351 = while {
        tunnel: w31 -> [w37]
        stop <- w38 stop-if-true
        n352 = event shown="[1] \"Scan\": Value Change" {
          selector: _ -> [_ _ _]
          dyn-events: _ -> [_ _ _]
          timeout: _ -> [_ _ _]
          tunnel: [_ _ w286] -> w38
          tunnel: w37 -> [_ w74 _]
          event "Cooling", "Pumping", "Detection", "Experiment": Value Change {
            n353 = event-data() -> ("CtlRef"=w40:refnum<vi>, "NewVal"=w39:bool)  [unwired: 1 in, 4 out]
            n354 = case shown="True" w39 {
              tunnel: w40 -> [_ w44]
              frame False {
              }
              frame True {
                n355 = flat-sequence {
                  tunnel: w44 -> [w46]
                  tunnel: [w46] -> w42
                  tunnel: w42 -> [w47]
                  tunnel: [w47] -> w41
                  tunnel: [w58] -> w43
                  tunnel: w41 -> [w56]
                  tunnel: w43 -> [w73]
                  frame #0 {
                    n356 = local write "Sweep"(FALSE ("Sweep")) -> ()
                  }
                  frame #1 {
                    n357 = while {
                      stop <- w49 continue-if-true
                      n358 = Wait (ms)(milliseconds to wait=u32 50) -> ()  [unwired: 1 out]
                      n359 = local read "Data"() -> (w49:bool)
                    }
                  }
                  frame #2 {
                    n360 = local read "Device"() -> (w52:string)
                    n361 = case shown="\"PMT\", Default" w52 {
                      tunnel: ["C" ("string") _] -> w50
                      frame "CCD" {
                      }
                      frame "PMT", Default {
                      }
                    }
                    n362 = property class="Bool (strict)"(reference=w56) -> (reference out=w58:refnum<vi>, "BoolText.Text"=w54:string)  [unwired: 1 in, 1 out]
                    n363 = Concatenate Strings(w54, w50, ".seq" ("string")) -> (w55:string)
                    n364 = Build Path(base path=path "E:/Data/Sequence", name or relative path=w55) -> (appended path=w53:path)
                    n365 = case shown="Default" w54 {
                      tunnel: w53 -> [w60 w62]
                      frame Default {
                        n366 = property on="Sequence File" class="Path"("Val(Sgnl)"=w60) -> ()  [unwired: 2 in, 2 out]
                      }
                      frame "Cooling", "Detection", "Pumping" {
                        n367 = flat-sequence {
                          tunnel: w62 -> [w64]
                          tunnel: [w64] -> w61
                          tunnel: w61 -> [w69]
                          frame #0 {
                            n368 = local read "Sequence File"() -> (w67:path)
                            n369 = Strip Path(path=w67) -> (name=w66:string)  [unwired: 1 out]
                            n370 = Search/Split String(string=w66, search string/char (-)=".") -> (substring before match=w63:string)  [unwired: 1 in, 2 out]
                            n371 = case shown="Default" w63 {
                              tunnel: w63 -> [_ w68]
                              frame "Cooling", "Detection", "Pumping" {
                              }
                              frame Default {
                                n372 = property on="Experiment" class="Bool (strict)"("BoolText.Text"=w68) -> ()  [unwired: 2 in, 2 out]
                              }
                            }
                          }
                          frame #1 {
                            n373 = property on="Sequence File" class="Path"("Val(Sgnl)"=w69) -> ()  [unwired: 2 in, 2 out]
                          }
                          frame #2 {
                            n374 = Wait (ms)(milliseconds to wait=u32 300) -> ()  [unwired: 1 out]
                          }
                          frame #3 {
                            n375 = property on="Sweep" class="Bool (strict)"("Val(Sgnl)"=TRUE ("Value (Signaling)")) -> ()  [unwired: 2 in, 2 out]
                          }
                        }
                      }
                    }
                  }
                  frame #3 {
                    n376 = property class="Bool (strict)"(reference=w73, "Value"=FALSE) -> ()  [unwired: 1 in, 2 out]
                  }
                }
              }
            }
          }
          event "Scan": Value Change {
            n377 = event-data() -> ("NewVal"=w75:bool)  [unwired: 1 in, 5 out]
            n378 = case shown="True" w75 {
              tunnel: w74 -> [w91 _]
              frame True {
                n379 = local read "Item"() -> (w93:string)
                n380 = Concatenate Strings(w93, "Scan-" ("string")) -> (w92:string)
                n381 = local read "Start"() -> (w102:dbl)
                n382 = flat-sequence {
                  tunnel: w92 -> [w108]
                  tunnel: w102 -> [w109]
                  tunnel: "Step" -> [w110]
                  tunnel: "End" -> [w111]
                  tunnel: w93 -> [w112]
                  tunnel: [w112] -> w87
                  tunnel: [w111] -> w85
                  tunnel: [w110] -> w83
                  tunnel: [w109] -> w81
                  tunnel: [w108] -> w79
                  tunnel: w91 -> [w107]
                  tunnel: [w106] -> w77
                  tunnel: w87 -> [w119]
                  tunnel: [w119] -> w86
                  tunnel: w85 -> [w118]
                  tunnel: [w118] -> w84
                  tunnel: w83 -> [w117]
                  tunnel: [w117] -> w82
                  tunnel: w81 -> [w116]
                  tunnel: [w116] -> w80
                  tunnel: w79 -> [w115]
                  tunnel: [w115] -> w78
                  tunnel: w77 -> [w114]
                  tunnel: [w114] -> w76
                  tunnel: [w137] -> w100
                  tunnel: [w126] -> w99
                  tunnel: [w131] -> w98
                  tunnel: [w130] -> w97
                  tunnel: [w129] -> w96
                  tunnel: [w128] -> w95
                  tunnel: w86 -> [w137]
                  tunnel: w84 -> [w134]
                  tunnel: w82 -> [w128]
                  tunnel: w80 -> [w129]
                  tunnel: w78 -> [w138]
                  tunnel: [w120] -> w89
                  tunnel: w76 -> [w120]
                  tunnel: [w177] -> w101
                  tunnel: w100 -> [w177]
                  tunnel: w99 -> [w183]
                  tunnel: w98 -> [w182]
                  tunnel: w97 -> [w181]
                  tunnel: w96 -> [w180]
                  tunnel: w95 -> [w179]
                  tunnel: [w178] -> w94
                  tunnel: [w176] -> w90
                  tunnel: w89 -> [w176]
                  tunnel: w101 -> [w280]
                  tunnel: w94 -> [w275]
                  tunnel: w90 -> [w273]
                  tunnel: [w273] -> w88
                  tunnel: w88 -> [w285]
                  frame #0 {
                    n383 = call "SequencerInitRS232.vi"("VISA resource name"=w107) -> ("reference out"=w106:refnum<visa-resource-name>)  [unwired: 1 out]
                  }
                  frame #1 {
                    n384 = Wait (ms)(milliseconds to wait=u32 200) -> ()  [unwired: 1 out]
                  }
                  frame #2 {
                    w142 = "\r\n"
                    n385 = Subtract(x=w134, y=w129) -> (x-y=w133:dbl)
                    n386 = local read "Parameter"() -> (w125:u16)
                    n387 = property on="Average Plot" class="WFChart (strict)"() -> ("History Data"=w124:cluster{dbl, dbl}[])  [unwired: 2 in, 2 out]
                    n388 = Divide(x=w133, y=w128) -> (x/y=w132:dbl)
                    n389 = case shown="Default" w137 {
                      tunnel: ["us" ("string") w165] -> w136
                      tunnel: [w156 w173] -> w135
                      tunnel: w125 -> [w152 w169]
                      frame "Time" {
                        n390 = local read "Durations"() -> (w163:dbl[])
                        n391 = local write "Durations Backup"(w163) -> ()
                        n392 = local read "Chapter (us)"() -> (w161:string)
                        n393 = local read "Sequence"() -> (w160:string)
                        n394 = call "SaveSequenceString.vi"("Sequence"=w160, "Chapter"=w161) -> ("Sequence String"=w158:string)
                        n395 = Number To Decimal String(number=w152) -> (decimal integer string=w154:string)  [unwired: 1 in]
                        n396 = Concatenate Strings("Sequence=\n{\n" ("string"), w158, "\n}\n" ("string"), "Index=" ("string"), w154, "\r\n") -> (w156:string)
                      }
                      frame Default {
                        w171 = u32 2 items=["Open", "Close", "Begin", "End", "Get", "Set"] ("Mode")
                        n397 = local read "Item Function"() -> (w170:refnum<vi>)
                        n398 = call-by-ref "?"(reference=w170, "In"=w169, "Mode"=w171) -> ("Out"=w168:variant)  [unwired: 1 in, 2 out]
                        n399 = Variant To Data(type=string[] [] ("Strings []"), Variant=w168) -> (data=w166:string[])  [unwired: 1 in, 1 out]
                        n400 = property on="Parameter" class="Ring (strict)"() -> ("RingText.Text"=w172:string)  [unwired: 2 in, 2 out]
                        n401 = Index Array(array=w166) -> (element #1=w165:string, element #2=w164:string)  [unwired: 2 in]
                        n402 = Concatenate Strings("Parameter=" ("string"), w172, "\r\n", w164) -> (w173:string)
                      }
                    }
                    n403 = Round Toward -Infinity(1:w132) -> (0:w127:dbl)
                    n404 = Array Subset(array=w124, length=0) -> (w122:cluster{dbl, dbl}[])  [unwired: 1 in]
                    n405 = property on="Average Plot" class="WFChart (strict)"("History Data"=w122, "XScale.Multiplier"=w128, "XScale.Offset"=w129, "XScale.Maximum"=w134) -> ()  [unwired: 2 in, 2 out]
                    n406 = To Unsigned Long Integer(number=w127) -> (unsigned 32bit integer=w126:u32)
                    n407 = call <vilib>:"Space Constant.vi"() -> ("String"=w141:string)
                    n408 = Concatenate Strings(w141, w136) -> (w131:string)
                    n409 = Number To Fractional String(number=w134) -> (F-format string=w147:string)  [unwired: 3 in]
                    n410 = Number To Fractional String(number=w128) -> (F-format string=w145:string)  [unwired: 3 in]
                    n411 = Number To Fractional String(number=w129) -> (F-format string=w149:string)  [unwired: 3 in]
                    n412 = call "NewData.vi"("Prefix"=w138, "data location"=path "E:/Data") -> ("data file name"=w139:string, "data file refnum"=w140:refnum<file>)  [unwired: 1 in]
                    n413 = local write "data file"(w139) -> ()
                    n414 = Concatenate Strings(w135, "Start=" ("string"), w149, w131, w142, "End=" ("string"), w147, w131, w142, "Step=" ("string"), w145, w131, w142, "Counts=" ("string"), w142, "{" ("string"), w142) -> (w150:string)
                    n415 = Write to Text File(file (use dialog)=w140, text=w150) -> (refnum out=w130:refnum<file>)  [unwired: 2 in, 2 out]
                  }
                  frame #3 {
                    n416 = while {
                      tunnel: w183 -> [w194]
                      tunnel: w182 -> [w190]
                      tunnel: w181 -> [w189]
                      shift-right: [w186] -> _
                      shift-left: w180 -> [w185]
                      tunnel: w179 -> [w188]
                      tunnel: [w187] -> w178
                      tunnel: w176 -> [w184]
                      i -> [w195]
                      stop <- w191 continue-if-true
                      n417 = flat-sequence {
                        tunnel: w185 -> [w196]
                        tunnel: w184 -> [w199]
                        tunnel: w190 -> [w261]
                        tunnel: w189 -> [w259]
                        tunnel: [w258] -> w187
                        tunnel: w185 -> [w257]
                        frame #0 {
                          n418 = local write "Value"(w196) -> ()
                        }
                        frame #1 {
                          n419 = property on="Set" class="Bool (strict)"("Val(Sgnl)"=TRUE ("Ready")) -> ()  [unwired: 2 in, 2 out]
                        }
                        frame #2 {
                          n420 = while {
                            stop <- w198 continue-if-true
                            n421 = local read "Set"() -> (w198:bool)
                          }
                        }
                        frame #3 {
                          n422 = while {
                            tunnel: w199 -> [w206]
                            stop <- w201 stop-if-true
                            n423 = flat-sequence {
                              tunnel: w206 -> [w210]
                              tunnel: [w210] -> w205
                              tunnel: [w209] -> w204
                              tunnel: w205 -> [w218]
                              tunnel: w204 -> [w217]
                              tunnel: [w215] -> w203
                              tunnel: [w245] -> w202
                              tunnel: w203 -> [w245]
                              tunnel: [w244] -> w200
                              frame #0 {
                                n424 = property on="Data" class="Bool (strict)"("Val(Sgnl)"=TRUE ("Value (Signaling)")) -> ()  [unwired: 2 in, 2 out]
                              }
                              frame #1 {
                                n425 = while {
                                stop <- w208 continue-if-true
                                n426 = local read "Data"() -> (w208:bool)
                                }
                              }
                              frame #2 {
                                w209 = u32 100 ("Repeats")
                                n427 = local read "Period (ns)"() -> (w214:dbl)
                                n428 = call "FPGAPackets.vi"("Repeats"=w209, "Period (ns)"=w214, "Durations"=dbl[] [1000.0, 1.0, 1.0, 10.0], "States"=string[] ["00000000000000000000000000001111", "00000000000000000000000000000000", "00000000000000000000000000010000", "10000000000000000000000000000000"]) -> ("Packets"=w211:string)  [unwired: 1 in, 1 out]
                                n429 = call "TxRS232.vi"("VISA resource name"=w210, "Data"=w211) -> ()
                              }
                              frame #3 {
                                n430 = local read "Device"() -> (w216:string)
                                n431 = case shown="\"PMT\", Default" w216 {
                                tunnel: w218 -> [_ w222]
                                tunnel: w217 -> [_ w232]
                                tunnel: [TRUE w223] -> w215
                                frame "CCD" {
                                }
                                frame "PMT", Default {
                                n432 = Multiply(x=w232, y=u32 4) -> (x*y=w231:u32)
                                n433 = Multiply(x=w231, y=3 ("Bytes To Read")) -> (x*y=w221:u32)
                                n434 = VISA Read(VISA resource name=w222, byte count=w221) -> (read buffer=w220:string)  [unwired: 1 in, 3 out]
                                n435 = for {
                                N: w231 -> [_]
                                tunnel: w220 -> [w243]
                                tunnel: [w234] -> w229 mode=indexing
                                i -> [w237]
                                w236 = 3 ("length (rest)")
                                n436 = Multiply(x=w237, y=w236) -> (x*y=w235:i32)
                                n437 = String Subset(string=w243, offset (0)=w235, length (rest)=w236) -> (substring=w238:string)
                                n438 = Concatenate Strings("\u0000" ("string"), w238) -> (w242:string)
                                n439 = To Unsigned Long Integer(number=u32 0) -> (unsigned 32bit integer=w239:u32)
                                n440 = Type Cast(type=w239, x=w242) -> (*(type *) &x=w234:u32)
                                }
                                n441 = Decimate 1D Array(w229) -> (w227:u32[])  [unwired: 3 out]
                                n442 = Add Array Elements(numeric array=w227) -> (sum=w228:u32)
                                n443 = Array Size(array=w227) -> (size(s)=w226:i32)
                                n444 = Divide(x=w228, y=w226) -> (x/y=w225:dbl)
                                n445 = Greater?(x=w225, y=2.0) -> (0:w223:bool)
                                }
                                }
                              }
                              frame #4 {
                                n446 = case shown="False" w245 {
                                selector: w245 -> [w247 w256]
                                tunnel: [w246 FALSE] -> w244
                                frame False {
                                n447 = flat-sequence {
                                tunnel: w247 -> [w248]
                                tunnel: [w249] -> w246
                                frame #0 {
                                n448 = property on="Ion" class="Bool (strict)"("Val(Sgnl)"=w248) -> ()  [unwired: 2 in, 2 out]
                                }
                                frame #1 {
                                n449 = while {
                                tunnel: [w250] -> w249
                                stop <- w251 stop-if-true
                                n450 = local read "Scan"() -> (w252:bool)
                                n451 = Wait (ms)(milliseconds to wait=u32 1000) -> ()  [unwired: 1 out]
                                n452 = Not(x=w252) -> (.not. x?=w250:bool)
                                n453 = local read "Ion"() -> (w253:bool)
                                n454 = Or(x=w253, y=w250) -> (x .or. y?=w251:bool)
                                }
                                }
                                }
                                }
                                frame True {
                                n455 = local write "Ion"(w256) -> ()
                                }
                                }
                              }
                            }
                            n456 = Or(x=w202, y=w200) -> (x .or. y?=w201:bool)
                          }
                        }
                        frame #4 {
                          n457 = Number To Fractional String(number=w257) -> (F-format string=w267:string)  [unwired: 3 in]
                          n458 = local read "Counts"() -> (w262:u32[])
                          n459 = Concatenate Strings(w267, w261, "," ("string")) -> (w266:string)
                          n460 = for {
                            tunnel: w262 -> [w272] mode=indexing
                            shift-right: [w270] -> w263
                            shift-left: w266 -> [w269]
                            n461 = Number To Decimal String(number=w272) -> (decimal integer string=w271:string)  [unwired: 1 in]
                            n462 = call <vilib>:"Space Constant.vi"() -> ("String"=w268:string)
                            n463 = Concatenate Strings(w269, w268, w271) -> (w270:string)
                          }
                          n464 = Concatenate Strings(w263, "\r\n") -> (w264:string)
                          n465 = Write to Text File(file (use dialog)=w259, text=w264) -> (refnum out=w258:refnum<file>)  [unwired: 2 in, 2 out]
                        }
                      }
                      n466 = Add(x=w185, y=w188) -> (x+y=w186:dbl)
                      n467 = Less?(x=w195, y=w194) -> (x < y?=w193:bool)
                      n468 = local read "Scan"() -> (w192:bool)
                      n469 = And(x=w193, y=w192) -> (x .and. y?=w191:bool)
                    }
                  }
                  frame #4 {
                    n470 = case shown="\"Time\"" w280 {
                      frame "Time" {
                        n471 = local read "Durations Backup"() -> (w281:dbl[])
                        n472 = local write "Durations"(w281) -> ()
                      }
                      frame Default {
                        w284 = u32 3 items=["Open", "Close", "Begin", "End", "Get", "Set"] ("Mode")
                        n473 = local read "Item Function"() -> (w283:refnum<vi>)
                        n474 = local read "Parameter"() -> (w282:u16)
                        n475 = call-by-ref "?"(reference=w283, "In"=w282, "Mode"=w284) -> ()  [unwired: 1 in, 3 out]
                      }
                    }
                    n476 = local write "Scan"(FALSE ("Scan")) -> ()
                    n477 = Concatenate Strings("}" ("string"), "\r\n") -> (w276:string)
                    n478 = Write to Text File(file (use dialog)=w275, text=w276) -> (refnum out=w279:refnum<file>)  [unwired: 2 in, 2 out]
                    n479 = Close File(refnum=w279) -> ()  [unwired: 1 in, 2 out]
                  }
                  frame #5 {
                    n480 = VISA Close(VISA resource name=w285) -> ()  [unwired: 1 in, 1 out]
                  }
                }
              }
              frame False, Default {
              }
            }
          }
          event "Sequencer": Value Change {
            n481 = event-data() -> ("NewVal"=w287:bool)  [unwired: 1 in, 5 out]
            n482 = flat-sequence {
              tunnel: [w289] -> w288
              tunnel: w287 -> [w289]
              tunnel: w288 -> [w292]
              tunnel: [w292] -> w286
              frame #0 {
                n483 = local write "Scan"(FALSE ("Scan")) -> ()
                n484 = local write "Sweep"(FALSE ("Sweep")) -> ()
              }
              frame #1 {
                n485 = property on="Data" class="Bool (strict)"("Val(Sgnl)"=FALSE ("Value (Signaling)")) -> ()  [unwired: 2 in, 2 out]
              }
            }
          }
        }
      }
    }
    frame #2 {
      n486 = local read "Port"() -> (w804:refnum<visa-resource-name>)
      n487 = VISA Close(VISA resource name=w804) -> ()  [unwired: 1 in, 1 out]
    }
  }
